vi "DoOperationPreview.vi"(8 "error in (no error)":errorcluster, 9 "Operator":enum16{"Add", "Divide", "Multiple", "Subtract"}(ring), 10 "TestStand UI ExpressionEdit Control 2":refnum<k7>, 11 "TestStand UI ExpressionEdit Control":refnum<k7>) -> (0 "error out":errorcluster, 3 "Result":dbl)   [LabVIEW 2013]
uses:
  ClassDefinitions/SimpleClassWithMethods/SimpleArithmetic.lvclass
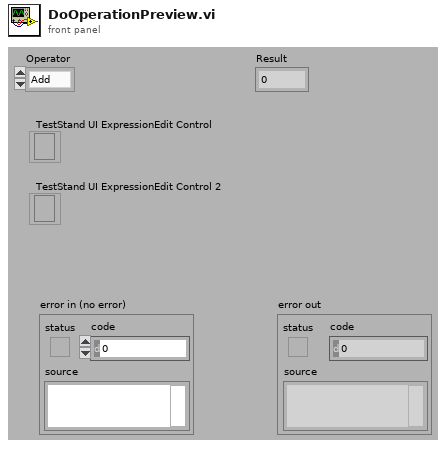
[diagram p1: front panel]
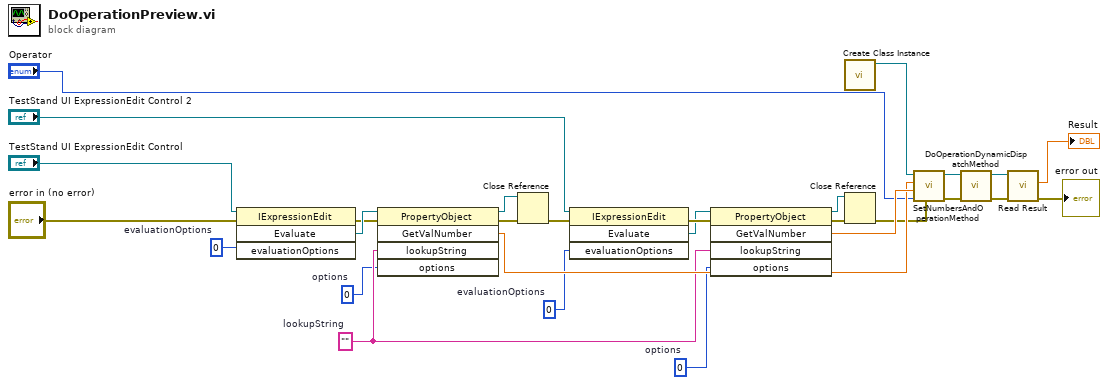
[diagram p0: block diagram]
diagram:
  w13 = 0  # options
  w14 = 0  # options
  w15 = ""  # lookupString
  w16 = 0  # evaluationOptions
  w17 = 0  # evaluationOptions
  n1 = invoke class="IExpressionEdit" method="Evaluate"(reference="TestStand UI ExpressionEdit Control", error in="error in (no error)", "evaluationOptions"=w16) -> (error out=w25:errorcluster, "Evaluate"=w26:refnum<k7>)  [unwired: 1 in, 2 out]
  n2 = invoke class="PropertyObject" method="GetValNumber"(reference=w26, error in=w25, "lookupString"=w15, "options"=w14) -> (reference out=w11:refnum<k7>, error out=w12:errorcluster, "GetValNumber"=w27:dbl)  [unwired: 1 in, 2 out]
  n3 = Close Reference(reference=w11, error in (no error)=w12) -> (error out=w3:errorcluster)
  n4 = invoke class="IExpressionEdit" method="Evaluate"(reference="TestStand UI ExpressionEdit Control 2", error in=w3, "evaluationOptions"=w17) -> (error out=w24:errorcluster, "Evaluate"=w22:refnum<k7>)  [unwired: 1 in, 2 out]
  n5 = invoke class="PropertyObject" method="GetValNumber"(reference=w22, error in=w24, "lookupString"=w15, "options"=w13) -> (reference out=w9:refnum<k7>, error out=w10:errorcluster, "GetValNumber"=w28:dbl)  [unwired: 1 in, 2 out]
  n6 = call "Create Class Instance.vi"() -> ("SimpleArithmetic.lvclass"=w19:refnum<class "SimpleArithmetic.lvclass">)  [unwired: 11 in]
  n7 = Close Reference(reference=w9, error in (no error)=w10) -> (error out=w2:errorcluster)
  n8 = call "SetNumbersAndOperationMethod.vi"("error in (no error)"=w2, "Operator"="Operator", "Numeric 2"=w28, "Numeric"=w27, "SimpleArithmetic in"=w19) -> ("error out"=w6:errorcluster, "SimpleArithmetic out"=w8:refnum<class "SimpleArithmetic.lvclass">)  [unwired: 5 in]
  n9 = call-dynamic "DoOperationDynamicDispatchMethod.vi"("error in (no error)"=w6, "SimpleArithmetic in"=w8) -> ("error out"=w5:errorcluster, "SimpleArithmetic out"=w7:refnum<class "SimpleArithmetic.lvclass">)  [unwired: 8 in]
  n10 = call "Read Result.vi"("error in (no error)"=w5, "SimpleArithmetic in"=w7) -> ("error out"=→"error out":errorcluster, "Result"=→"Result":dbl)  [unwired: 7 in, 1 out]
